vi "test_srv.vi"   [LabVIEW 2012]
uses:
  <vilib>/Platform/TimedLoop/XDataNode/XDataNode.xnode
  <vilib>/Platform/TimedLoop/XDataNode/nitl_modes.ctl
  <vilib>/Platform/TimedLoop/XDataNode/XDNodeRunTimeDep.lvlib
  <vilib>/Platform/TimedLoop/XDataNode/wakeup.ctl
  <vilib>/Platform/TimedLoop/XDataNode/timing_clust.ctl
types:
  T1 = enum16{"set date", "set local time", "set UTC time"}
  T2 = typedef "LVDateTimeRec.ctl" = cluster{"fractional second":dbl, "second":i32, "minute":i32, "hour":i32, "day of month":i32, "month":i32, "year":i32, "day of week":i32, "day of year":i32, "DST":i32}
  T3 = cluster{"month":i32, "day of month":i32, "year":i32}
  T4 = typedef "XDNodeRunTimeDep.lvlib/timing_clust.ctl" = cluster{"Expected End [f-1]":u64, "Actual End [f-1]":u64, "Finished Late? [f-1]":bool, "Expected End [i-1]":u64, "Actual End [i-1]":u64, "Finished Late? [i-1]":bool, "Expected Start [i]":u64, "Actual Start [i]":u64, "Expected Start [f]":u64, "Actual Start [f]":u64, "Source Name":string, "Structure Name":string, "Period":i64, "Deadline":i64, "Offset":i64, "Start":i64, "Priority":i32, "Timeout":i32, "Mode":T5, "Wakeup Reason":T6, "Error":errorcluster, "Source Type":string, "Secondary Source Type":string, "Global End Time":u64, "Global Start Time":u64, "Frame Duration":u64, "Iteration Duration":u64, "Assigned CPU":i32, "I/O Scan Engine Mode":u32}
  T5 = typedef "XDNodeRunTimeDep.lvlib/nitl_modes.ctl" = enum32{"No Change", "Process missed periods, maintain original phase", "Discard missed periods, maintain original phase", "Process missed periods, ignore original phase", "Discard missed periods, ignore original phase"}
  T6 = typedef "XDNodeRunTimeDep.lvlib/wakeup.ctl" = enum32{"Normal", "Aborted", "Asynchronous wakeup", "Timing source error", "Timed loop error", "Timeout"}
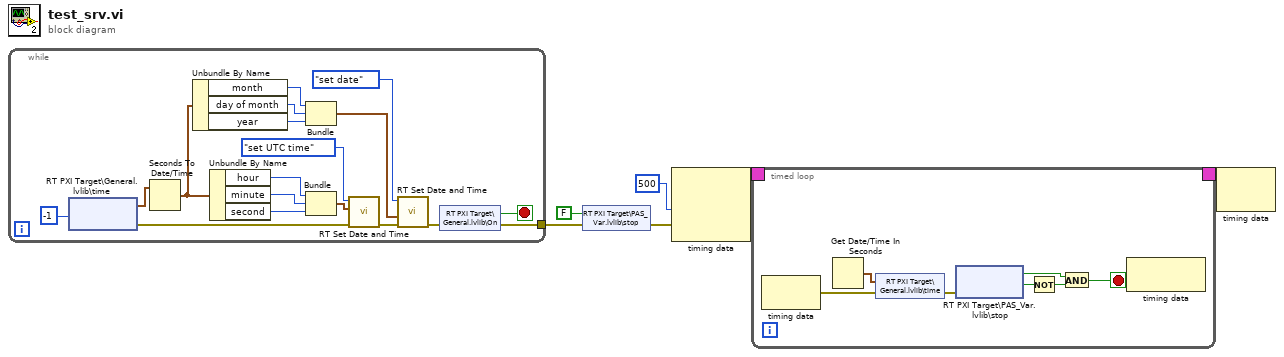
[diagram p0: block diagram]
diagram:
  n1 = while {
    tunnel: [w23] -> w2
    stop <- w24 stop-if-true
    n2 = shared-variable "RT PXI Target\\General.lvlib\\time"(-1 ("ms timeout (0)")) -> (w18:timestamp, error out=w7:errorcluster)  [unwired: 1 in, 1 out]
    n3 = Seconds To Date/Time(time stamp (now)=w18) -> (date time rec=w14:T2)  [unwired: 1 in]
    n4 = Unbundle By Name(w14) -> ("month"=w13:i32, "day of month"=w12:i32, "year"=w11:i32)
    n5 = Unbundle By Name(w14) -> ("hour"=w19:i32, "minute"=w20:i32, "second"=w21:i32)
    n6 = Bundle("month"=w13, "day of month"=w12, "year"=w11) -> (w10:T3)  [unwired: 1 in]
    n7 = Bundle("hour"=w19, "minute"=w20, "second"=w21) -> (w17:cluster{"hour":i32, "minute":i32, "second":i32})  [unwired: 1 in]
    n8 = call <vilib>:"RT Set Date and Time.vi"("error in (no error)"=w7, "Time"=w17, "mode"=T1."set UTC time") -> ("error out"=w16:errorcluster)  [unwired: 8 in]
    n9 = call <vilib>:"RT Set Date and Time.vi"("error in (no error)"=w16, "Date"=w10, "mode"=T1."set date") -> ("error out"=w8:errorcluster)  [unwired: 8 in]
    n10 = shared-variable "RT PXI Target\\General.lvlib\\On"(error in=w8) -> (w24:bool, error out=w23:errorcluster)
  }
  n11 = shared-variable "RT PXI Target\\PAS_Var.lvlib\\stop"(FALSE ("stop"), error in=w2) -> (error out=w1:errorcluster)
  n12 = node-c288(i64 500 ("Period"), w1) -> (w6:T4)  [unwired: 1 in]
  n13 = timed-loop {
    timing: w6 -> [_]
    timing-out: [_] -> w5
    stop <- w27 stop-if-true
    n14 = node-c288() -> (w25:errorcluster)  [unwired: 1 in]
    n15 = Get Date/Time In Seconds() -> (seconds since 1Jan1904=w31:timestamp)
    n16 = shared-variable "RT PXI Target\\General.lvlib\\time"(w31, error in=w25) -> (error out=w26:errorcluster)
    n17 = shared-variable "RT PXI Target\\PAS_Var.lvlib\\stop"(error in=w26) -> (w28:bool, w30:bool)  [unwired: 1 in, 1 out]
    n18 = Not(x=w30) -> (.not. x?=w29:bool)
    n19 = And(x=w28, y=w29) -> (x .and. y?=w27:bool)
    n20 = node-c288() -> ()  [unwired: 1 in, 1 out]
  }
  n21 = node-c288(w5) -> ()  [unwired: 1 out]
